vi "Node Contants.vi"(8 "error in (no error)":errorcluster) -> (0 "error out":errorcluster, 2 "Constants":T1)   [LabVIEW 2019, in "Picture Ring.lvclass"]
uses:
  Picture Ring.lvclass
  Node Type--enum.ctl
  Picture Ring.lvclass/Picture Ring.ctl
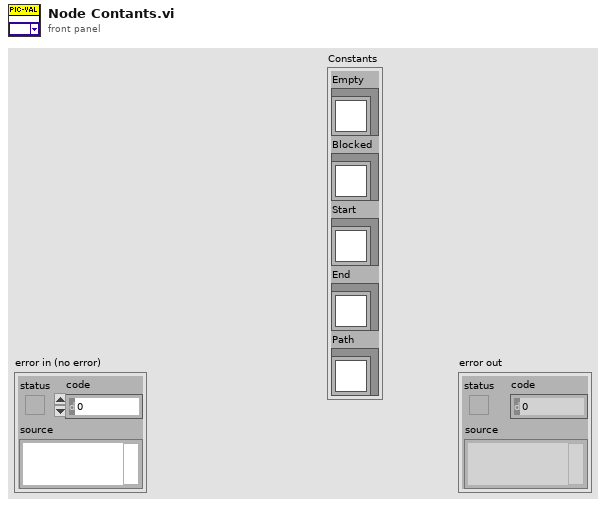
[diagram p1: front panel]
types:
  T1 = cluster{"Empty":refnum<class "Picture Ring.lvclass">, "Blocked":refnum<class "Picture Ring.lvclass">, "Start":refnum<class "Picture Ring.lvclass">, "End":refnum<class "Picture Ring.lvclass">, "Path":refnum<class "Picture Ring.lvclass">}
  T2 = typedef "Picture Ring.lvclass/Node Type--enum.ctl" = enum16{"Empty", "Blocked", "Start", "End", "Path"}
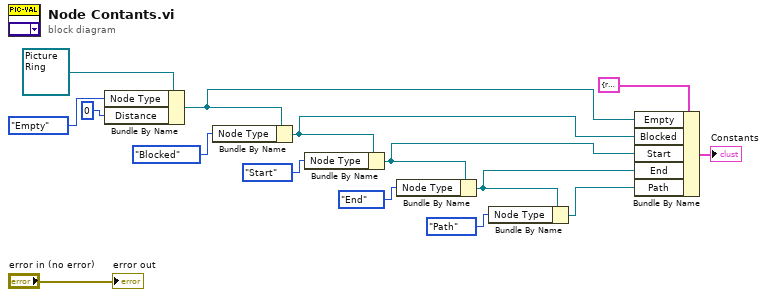
[diagram p0: block diagram]
diagram:
  n1 = Bundle By Name(cluster=refnum<class "Picture Ring.lvclass"> refnum ("Picture Ring.lvclass"), "Node Type"=Node_Type--enum."Empty", "Distance"=0) -> (w7:refnum<class "Picture Ring.lvclass">)
  n2 = Bundle By Name(cluster=w7, "Node Type"=Node_Type--enum."Blocked") -> (w6:refnum<class "Picture Ring.lvclass">)
  n3 = Bundle By Name(cluster=w6, "Node Type"=Node_Type--enum."Start") -> (w5:refnum<class "Picture Ring.lvclass">)
  n4 = Bundle By Name(cluster=w5, "Node Type"=Node_Type--enum."End") -> (w4:refnum<class "Picture Ring.lvclass">)
  n5 = Bundle By Name(cluster=w4, "Node Type"=Node_Type--enum."Path") -> (w3:refnum<class "Picture Ring.lvclass">)
  n6 = Bundle By Name(cluster=T1 {"Empty"=refnum, "Blocked"=refnum, "Start"=refnum, "End"=refnum, "Path"=refnum} ("Constants"), "Empty"=w7, "Blocked"=w6, "Start"=w5, "End"=w4, "Path"=w3) -> (→"Constants":T1)
  "error out" <- "error in (no error)"
